vi "Set Version Number.vi"(8 "error in (no error)":errorcluster, 10 "Version number":T1, 11 "EXE in":refnum<class "NI_AB_API_EXE.lvclass">) -> (0 "error out":errorcluster, 3 "EXE out":refnum<class "NI_AB_API_EXE.lvclass">)   [LabVIEW 2020, in "NI_AB_API_EXE.lvclass"]
uses:
  <vilib>/AppBuilder/AB_API/EXE/NI_AB_API_EXE.lvclass
  <vilib>/AppBuilder/AB_API/common/AB_API Version Number.ctl
  <vilib>/AppBuilder/AB_API/Application/NI_AB_API_Application.lvclass
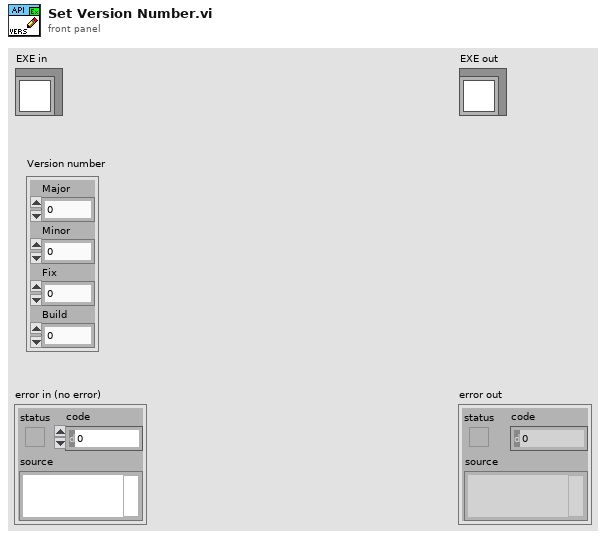
[diagram p1: front panel]
types:
  T1 = typedef "AB_API Version Number.ctl" = cluster{"Major":u16, "Minor":u16, "Fix":u16, "Build":u16}
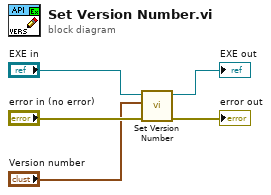
[diagram p0: block diagram]
diagram:
  n1 = call-parent "Set Version Number.vi"("error in (no error)"="error in (no error)", "Version number"="Version number", "NI_AB_API_Targetfile in"="EXE in") -> ("error out"=→"error out":errorcluster, "NI_AB_API_Targetfile out"=→"EXE out":refnum<class "NI_AB_API_EXE.lvclass">)  [unwired: 7 in]
